vi "Test Cast.vi"() -> ()   [LabVIEW 2014, in "Meerstetter Lib.lvlib" / "Meerstetter TEC.lvclass"]
uses:
  Meerstetter TEC.lvclass
  Driver/Controls/Ctl Method.ctl
panel:
  in  "String":string="Power"
  out "Typecast":T1
  out "Scan from Str":T1
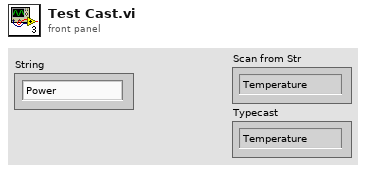
[diagram p1: front panel]
types:
  T1 = typedef "Ctl Method.ctl" = enum16{"Temperature", "Power"}
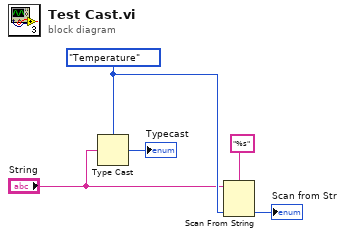
[diagram p0: block diagram]
diagram:
  w5 = Ctl_Method."Temperature" ("ctlVal")
  n1 = Type Cast(type=w5, x="String") -> (*(type *) &x=→"Typecast":T1)
  n2 = Scan From String(format string="%s", input string="String", default 1=w5) -> (output 1=→"Scan from Str":T1)  [unwired: 2 in, 3 out]
